vi "Add State(s) to Queue By BOOL(Array Right).vi"(4 "False(\"\")":string[](array[string]), 6 "TRUE(\"\")":string, 8 "High Priority(FALSE)":bool, 10 "Bool":bool, 11 "State Queue(\"\")":string) -> (3 "State Queue Out":string)   [LabVIEW 2014, in "JKI State Machine++.lvlib"]
doc: "根据高优先级和Bool输入，此VI生成TRUE/False和剩余状态的连接状态。High Priority输入决定是否在剩余状态之前或之后连接TRUE或False字符串。Bool输入决定要连接的字符串是TRUE还是False。\n\n<b>Inputs:</b>\n - <b>State Queue(\"\")</b>: 整个状态队列被连接到此输入\n - <b>TRUE(\"\")</b>: <b>Bool</b> 为 True 时插入的状态字符串\n - <b>False(\"\")</b>: <b>Bool</b> 为 False 时插入的状态字符串\n - <b>Bool</b>: 选择连接到TRUE终端或False终端的状态字符串的标志。\n - <b>High Priority(FALSE)</b>: 如果为True，状态将被插入到<b>State Queue(\"\")</b>的顶部。如果为False，它被附加到尾部。\n\n<b>Outputs:</b>\n - <b>State Queue Out</b>: 返回继续执行的所有状态及参数。"
uses:
  JKI State Machine++.lvlib
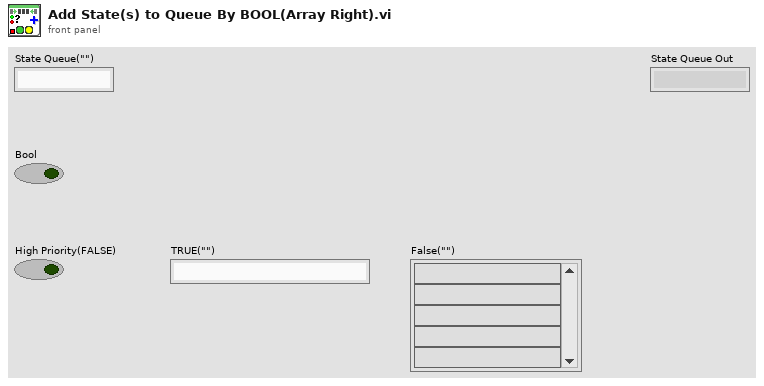
[diagram p1: front panel]
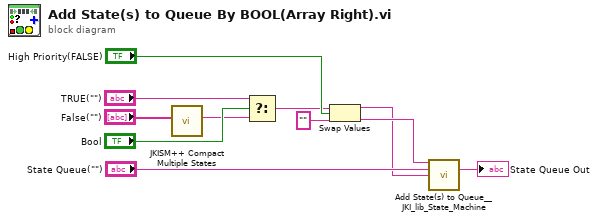
[diagram p0: block diagram]
diagram:
  n1 = call "JKISM++ Compact Multiple States.vi"("States in Lines"="False(\"\")") -> ("States"=w1:string)  [unwired: 9 in]
  n2 = Select(t="TRUE(\"\")", s="Bool", f=w1) -> (s? t:f=w5:string)
  n3 = Swap Values(12:w5, 13:"High Priority(FALSE)", 14:"") -> (1:w2:string, 3:w3:string)
  n4 = call <vilib>:"Add State(s) to Queue__JKI_lib_State_Machine.vi"("State(s) in Front (\"\")"=w3, "State(s) in (\"\")"="State Queue(\"\")", "State(s) at Back (\"\")"=w2) -> ("States Out"=→"State Queue Out":string)  [unwired: 12 in]
